vi "Logging Split Path.vi"(0 "Path In":string) -> (1 "Name":string, 2 "Split Path":string[](array[string]))   [LabVIEW 2012, in "femtoRoboLib.lvlib"]
uses:
  femtoRoboLib.lvlib
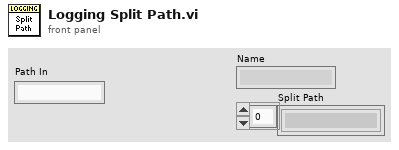
[diagram p1: front panel]
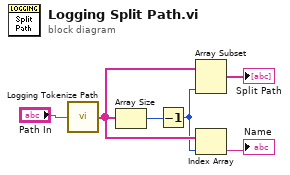
[diagram p0: block diagram]
diagram:
  n1 = call "Logging Tokenize Path.vi"("Name"="Path In") -> ("Array"=w4:string[])
  n2 = Array Size(array=w4) -> (size(s)=w5:i32)
  n3 = Decrement(x=w5) -> (x-1=w3:i32)
  n4 = Array Subset(array=w4, length=w3) -> (→"Split Path":string[])  [unwired: 1 in]
  n5 = Index Array(array=w4, index=w3) -> (element=→"Name":string)
